vi "Get Images.vi"(8 "error in (no error)":errorcluster, 11 "ParseSVG in":refnum<class "ParseSVG.lvclass">) -> (0 "error out":errorcluster, 3 "ParseSVG out":refnum<class "ParseSVG.lvclass">)   [LabVIEW 2019, in "ParseSVG.lvclass"]
uses:
  ParseSVG.lvclass
  Image.ctl
  ParseSVG.lvclass/ParseSVG.ctl
  Read RawXML.vi
  <userlib>/_OpenG.lib/lvdata/lvdata.llb/Get Data Name__ogtk.vi
  <userlib>/_OpenG.lib/lvdata/lvdata.llb/Get Cluster Element Names__ogtk.vi
  <userlib>/_OpenG.lib/lvdata/lvdata.llb/Array of VData to VCluster__ogtk.vi
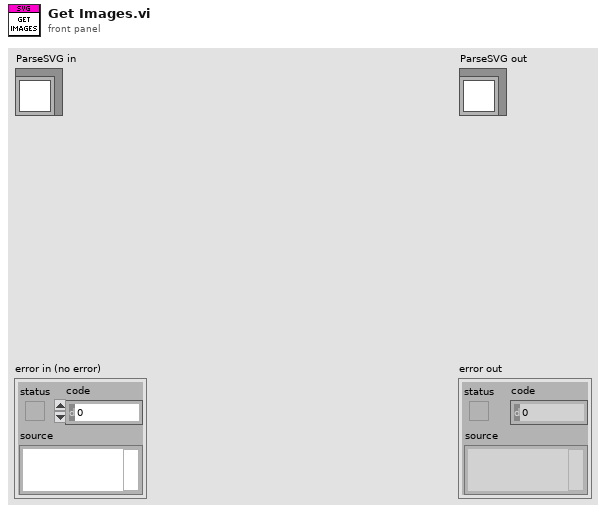
[diagram p1: front panel]
types:
  T1 = typedef "ParseSVG.lvclass/Image.ctl" = cluster{"x":string, "y":string, "width":string, "height":string, "xlink:href":string, "id":string, "transform":string}
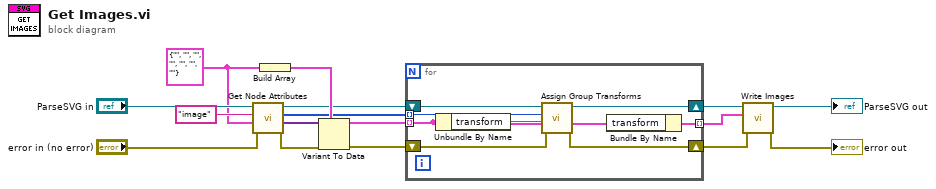
[diagram p0: block diagram]
diagram:
  w14 = T1 {"x"="", "y"="", "width"="", "height"="", "xlink:href"="", "id"="", "transform"=""} ("image")
  n1 = call "Get Node Attributes.vi"("error in (no error)"="error in (no error)", "Attributes Cluster"=w14, "Node Name (exact)"="image", "ParseSVG in"="ParseSVG in") -> ("error out"=w10:errorcluster, "[Attributes Cluster]"=w13:variant[], "Positions"=w7:i32[], "ParseSVG out"=w1:refnum<class "ParseSVG.lvclass">)  [unwired: 4 in]
  n2 = Build Array(w14) -> (w12:T1[])
  n3 = Variant To Data(error in=w10, type=w12, Variant=w13) -> (data=w6:T1[], error out=w5:errorcluster)
  n4 = for {
    shift-right: [w24] -> w3
    shift-left: w1 -> [w25]
    shift-right: [w22] -> w4
    shift-left: w5 -> [w23]
    tunnel: w6 -> [w19] mode=indexing
    tunnel: w7 -> [w20] mode=indexing
    tunnel: [w17] -> w2 mode=indexing
    n5 = Unbundle By Name(w19) -> ("transform"=w21:string)
    n6 = call "Assign Group Transforms.vi"("error in (no error)"=w23, "transform in"=w21, "position"=w20, "ParseSVG in"=w25) -> ("error out"=w22:errorcluster, "transform out"=w18:string, "ParseSVG out"=w24:refnum<class "ParseSVG.lvclass">)  [unwired: 5 in]
    n7 = Bundle By Name(cluster=w19, "transform"=w18) -> (w17:T1)
  }
  n8 = call "Write Images.vi"("error in (no error)"=w4, "Images"=w2, "ParseSVG in"=w3) -> ("error out"=→"error out":errorcluster, "ParseSVG out"=→"ParseSVG out":refnum<class "ParseSVG.lvclass">)  [unwired: 7 in]
